vi "pmu_Check Name Length CFG-3.vi"(8 "error in (no error)":errorcluster, 11 "name in":string) -> (0 "error out":errorcluster, 3 "name out":string)   [LabVIEW 2013, in "NI_EP_PMU.lvlib"]
uses:
  <vilib>/addons/Electrical Power/PMU/NI_EP_PMU.lvlib
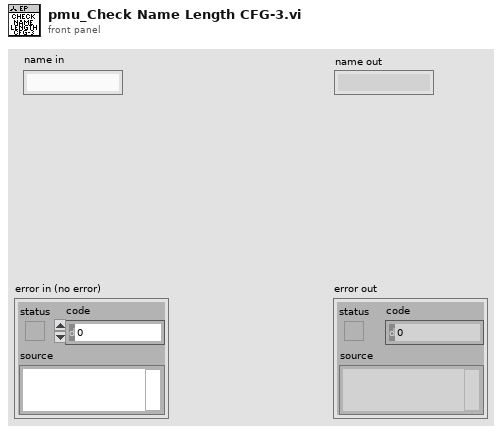
[diagram p1: front panel]
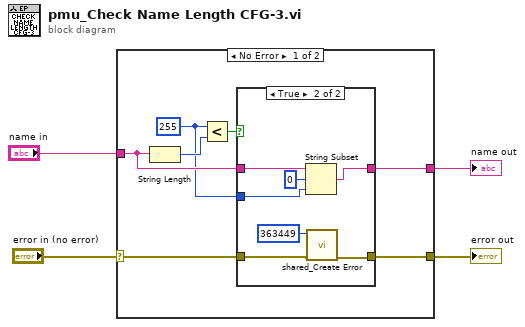
[diagram p0: block diagram]
diagram:
  n1 = case shown="No Error" "error in (no error)" {
    selector: "error in (no error)" -> [w10 w21]
    tunnel: [w9 w21] -> w3
    tunnel: "name in" -> [w7 _]
    tunnel: [w6 _] -> w1
    frame No Error {
      w5 = 255 ("y")
      n2 = String Length(string=w7) -> (length=w8:i32)
      n3 = Less?(x=w5, y=w8) -> (x < y?=w11:bool)
      n4 = case shown="True" w11 {
        tunnel: w10 -> [w13 w17]
        tunnel: [w13 w16] -> w9
        tunnel: w7 -> [w12 w20]
        tunnel: [w12 w19] -> w6
        tunnel: w5 -> [_ w14]
        frame False {
        }
        frame True {
          n5 = String Subset(string=w20, offset (0)=0, length (rest)=w14) -> (substring=w19:string)
          n6 = call <vilib>:"shared_Create Error.vi"("error in (no error)"=w17, "error code (0)"=363449) -> ("error out"=w16:errorcluster)  [unwired: 9 in]
        }
      }
    }
    frame Error {
    }
  }
  "error out" <- w3
  "name out" <- w1
